vi "JSON to LabVIEW.vi"(8 "error in (no error)":errorcluster, 9 "datatype and defaults":dbl, 10 "JSON Value in":refnum<class "JSON Value.lvclass">) -> (0 "error out":errorcluster, 3 "data":dbl)   [LabVIEW 2016]
uses:
  JSON Value.lvclass
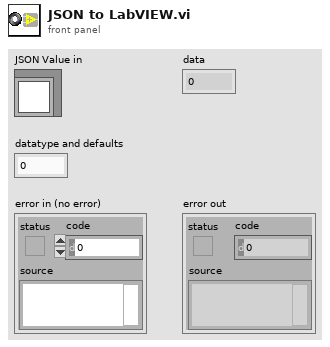
[diagram p1: front panel]
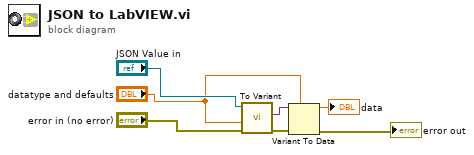
[diagram p0: block diagram]
diagram:
  n1 = call "To Variant.vi"("error in (no error)"="error in (no error)", "datatype and defaults"="datatype and defaults", "JSON Value in"="JSON Value in") -> ("error out"=w5:errorcluster, "Variant"=w4:variant)  [unwired: 6 in, 1 out]
  n2 = Variant To Data(error in=w5, type="datatype and defaults", Variant=w4) -> (data=→"data":dbl, error out=→"error out":errorcluster)
